vi "File Page - Set Stop Trigger.vi"(7 "File Ctl Refs":T3, 8 "error in (no error)":errorcluster, 10 "Stop Trigger":T1 caption="Trigger condition", 11 "Item Ref in":T2 format="%.0x") -> (0 "error out":errorcluster)   [LabVIEW 2015, in "Waveform Data Logger System Explorer.lvlib"]
uses:
  Waveform Data Logger System Explorer.lvlib
  Types/File Ctl Refs.ctl
  Types/File - Spec Ctl Refs.ctl
  Types/File - Wfm Ctl Refs.ctl
  Types/File - Settings Ctl Refs.ctl
  Classes/Log File Specifications/Log File Specification/File Conflict Operation.ctl
  Types/File - Start Trig Ctl Refs.ctl
  Shared/Types/Start Trigger.ctl
  Shared/Types/Default Trigger.ctl
  Shared/Types/Digital Trigger.ctl
  Shared/Types/Analog Trigger.ctl
  Shared/Types/In Range Trigger.ctl
  Shared/Types/Value Change Trigger.ctl
  Shared/Types/Boolean Trigger.ctl
  Types/Single Node Browser Data.ctl
  <vilib>/NI Veristand/UI Controls/Single Node Browser/Single Node Browser Ref.ctl
  NationalInstruments.VeriStand.SystemStorageUI
  <vilib>/NI Veristand/UI Controls/Single Node Browser/Callback Type.ctl
  <vilib>/NI Veristand/UI Controls/Single Node Browser/Net Event Data.ctl
  <vilib>/NI Veristand/UI Controls/Single Node Browser/Net Event.ctl
  Types/File - Stop Trig Ctl Refs.ctl
  Shared/Types/Stop Trigger.ctl
  Types/File - Advanced Ctl Refs.ctl
  Types/Log Timestamps.ctl
  <vilib>/NI Veristand/Custom Device API/Custom Device Item Ref.ctl
  NationalInstruments.VeriStand.SystemStorage
  Shared/Globals/Property Strings.vi
  <vilib>/NI Veristand/Custom Device API/Set Item Property (U16).vi
  <vilib>/NI Veristand/Custom Device API/Get Item Property (Dependent Node Pointer).vi
  <vilib>/NI Veristand/Custom Device API/Set Item Property (Dependent Node Pointer).vi
  <vilib>/NI Veristand/Custom Device API/Custom Device API.lvlib
  Shared/Waveform Data Logger Shared.lvlib
  Classes/Log File Specifications/Log File Specification/Log File Specification.lvclass
  <vilib>/NI Veristand/UI Controls/Single Node Browser/NI_VS UI Single Node Browser.lvlib
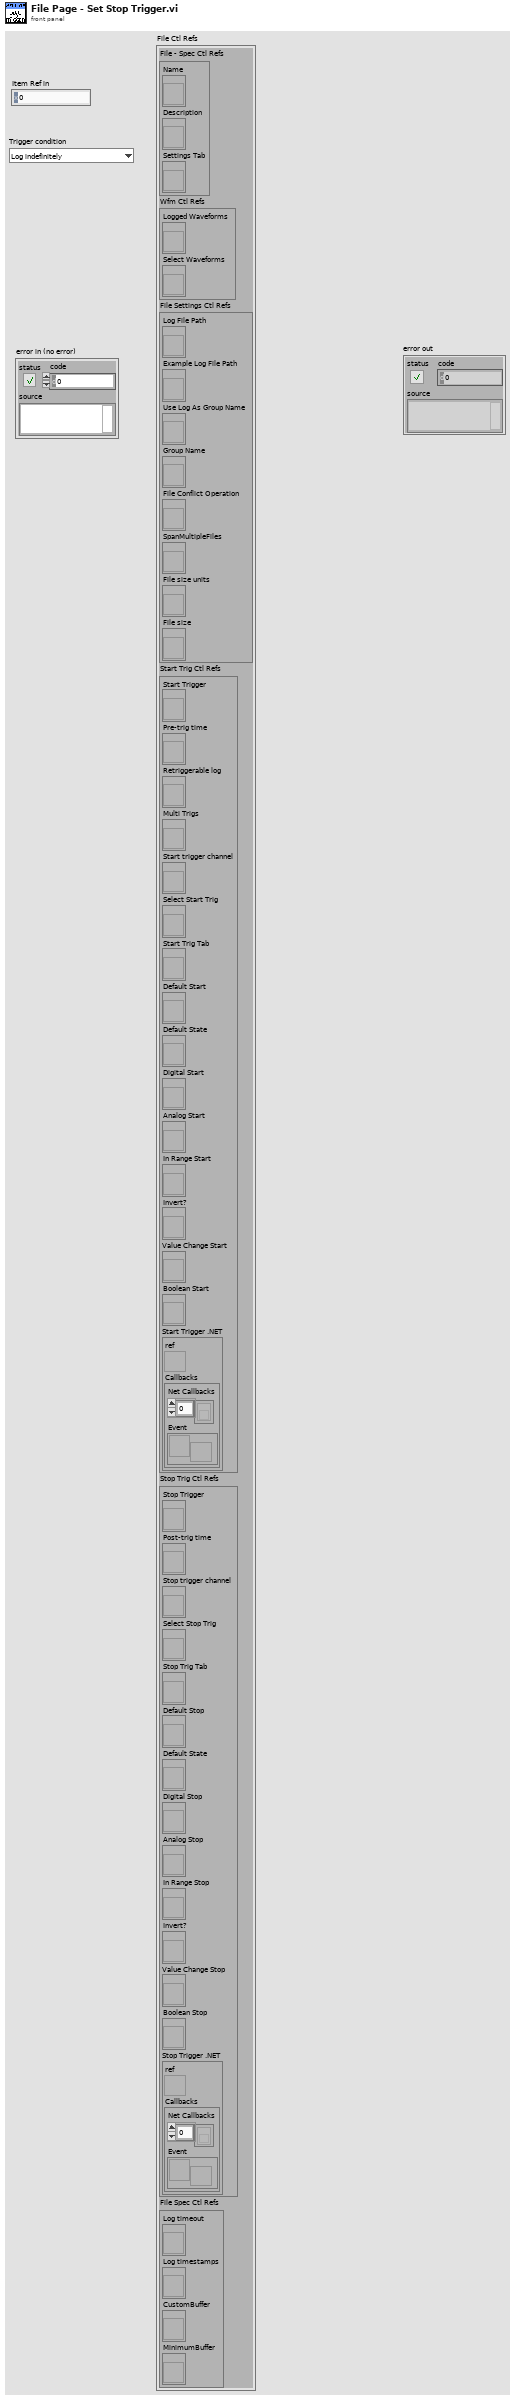
[diagram p1: front panel]
types:
  T1 = typedef "Waveform Data Logger Shared.lvlib/Stop Trigger.ctl" = enum16{"Log indefinitely", "Stop after duration", "Stop on digital edge", "Stop on analog edge", "Stop when in range", "Stop when out of range", "Stop on value change", "Stop when Boolean condition is true"}
  T2 = typedef "Custom Device API.lvlib/Custom Device Item Ref.ctl" = u64
  T3 = typedef "Waveform Data Logger System Explorer.lvlib/File Ctl Refs.ctl" = cluster{"File Spec Ctl Refs":T4, "Wfm Ctl Refs":T5, "File Settings Ctl Refs":T6, "Start Trig Ctl Refs":T7, "Stop Trig Ctl Refs":T11, "File Spec Ctl Refs":T12}
  T4 = typedef "Waveform Data Logger System Explorer.lvlib/File - Spec Ctl Refs.ctl" = cluster{"Name":refnum<vi>, "Description":refnum<vi>, "Settings Tab":refnum<vi>}
  T5 = typedef "Waveform Data Logger System Explorer.lvlib/File - Wfm Ctl Refs.ctl" = cluster{"Logged Waveforms":refnum<vi>, "Select Waveforms":refnum<vi>}
  T6 = typedef "Waveform Data Logger System Explorer.lvlib/File - Settings Ctl Refs.ctl" = cluster{"Log File Path":refnum<vi>, "Example Log File Path":refnum<vi>, "Use Log As Group Name":refnum<vi>, "Group Name":refnum<vi>, "File Conflict Operation":refnum<vi>, "SpanMultipleFiles":refnum<vi>, "File size units":refnum<vi>, "File size":refnum<vi>}
  T7 = typedef "Waveform Data Logger System Explorer.lvlib/File - Start Trig Ctl Refs.ctl" = cluster{"Start Trigger":refnum<vi>, "Pre-trig time":refnum<vi>, "Retriggerable log":refnum<vi>, "Multi Trigs":refnum<vi>, "Start trigger channel":refnum<vi>, "Select Start Trig":refnum<vi>, "Start Trig Tab":refnum<vi>, "Default Start":refnum<vi>, "Default State":refnum<vi>, "Digital Start":refnum<vi>, "Analog Start":refnum<vi>, "In Range Start":refnum<vi>, "Invert?":refnum<vi>, "Value Change Start":refnum<vi>, "Boolean Start":refnum<vi>, "Start Trigger .NET":T8}
  T8 = typedef "Waveform Data Logger System Explorer.lvlib/Single Node Browser Data.ctl" = cluster{"ref":T9, "Callbacks":T10}
  T9 = typedef "NI_VS UI Single Node Browser.lvlib/Single Node Browser Ref.ctl" = refnum<k24>
  T10 = typedef "NI_VS UI Single Node Browser.lvlib/Callback Type.ctl" = cluster{"Net Callbacks":refnum<k27>[], "Event":refnum<user-event>}
  T11 = typedef "Waveform Data Logger System Explorer.lvlib/File - Stop Trig Ctl Refs.ctl" = cluster{"Stop Trigger":refnum<vi>, "Post-trig time":refnum<vi>, "Stop trigger channel":refnum<vi>, "Select Stop Trig":refnum<vi>, "Stop Trig Tab":refnum<vi>, "Default Stop":refnum<vi>, "Default State":refnum<vi>, "Digital Stop":refnum<vi>, "Analog Stop":refnum<vi>, "In Range Stop":refnum<vi>, "Invert?":refnum<vi>, "Value Change Stop":refnum<vi>, "Boolean Stop":refnum<vi>, "Stop Trigger .NET":T8}
  T12 = typedef "Waveform Data Logger System Explorer.lvlib/File - Advanced Ctl Refs.ctl" = cluster{"Log timeout":refnum<vi>, "Log timestamps":refnum<vi>, "CustomBuffer":refnum<vi>, "MinimumBuffer":refnum<vi>}
  T13 = enum32{"Default", "Digital", "Analog", "In Range", "Value Change", "Boolean"}
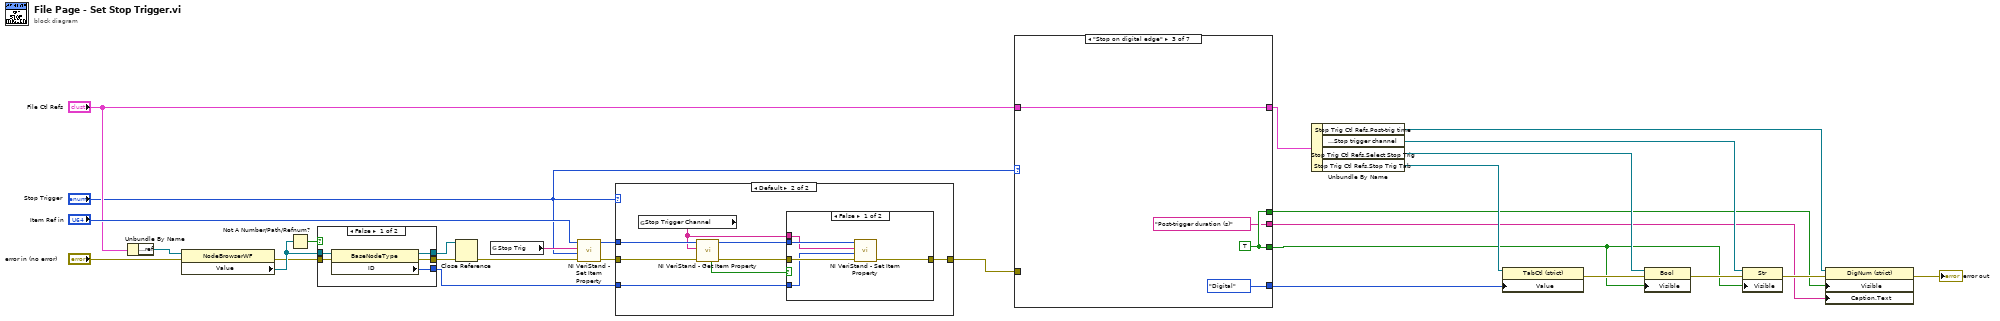
[diagram p0: block diagram]
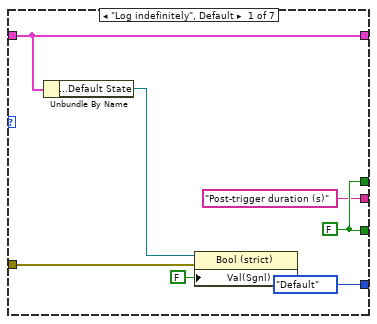
[diagram p2: hidden frame]
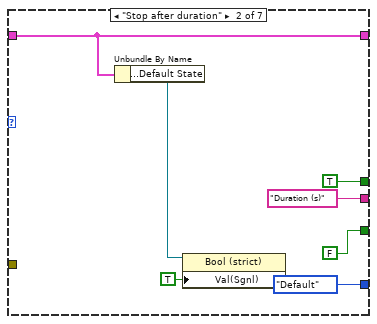
[diagram p3: hidden frame]
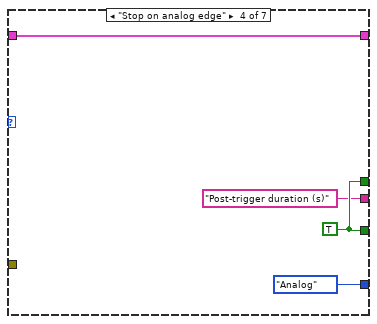
[diagram p4: hidden frame]
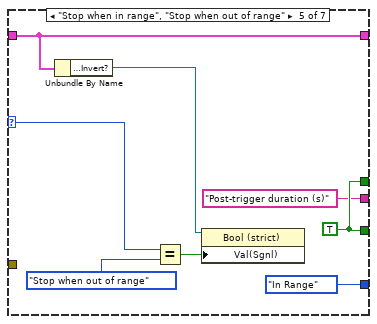
[diagram p5: hidden frame]
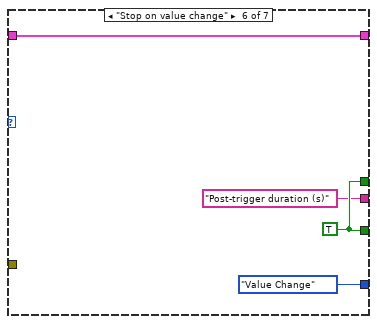
[diagram p6: hidden frame]
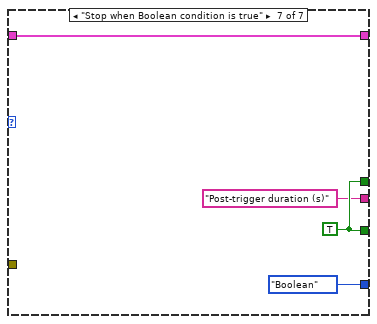
[diagram p7: hidden frame]
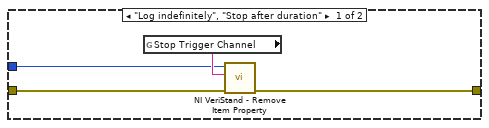
[diagram p8: hidden frame]
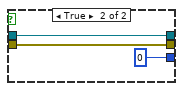
[diagram p10: hidden frame]
diagram:
  n1 = Unbundle By Name("File Ctl Refs") -> ("Stop Trig Ctl Refs.Stop Trigger .NET.ref"=w28:T9)
  n2 = property class="NodeBrowserWF"(reference=w28, error in="error in (no error)") -> (error out=w25:errorcluster, "Value"=w26:refnum<k24>)  [unwired: 1 out]
  n3 = Not A Number/Path/Refnum?(number/path/refnum=w26) -> (NaN/Path/Refnum?=w27:bool)
  n4 = case shown="False" w27 {
    tunnel: [w34 u64 0 ("ID")] -> w17
    tunnel: w25 -> [w33 w37]
    tunnel: [w30 w37] -> w24
    tunnel: w26 -> [w32 w35]
    tunnel: [w31 w35] -> w23
    frame False {
      n5 = property class="BaseNodeType"(reference=w32, error in=w33) -> (reference out=w31:refnum<k24>, error out=w30:errorcluster, "ID"=w34:u64)
    }
    frame True {
    }
  }
  n6 = Close Reference(reference=w23, error in (no error)=w24) -> (error out=w21:errorcluster)
  n7 = global read "Property Strings.vi" "Stop Trig"() -> (w22:string)
  n8 = call-poly <vilib>:"NI VeriStand - Set Item Property.vi"("error in (no error)"=w21, "Value"="Stop Trigger", "Property Name"=w22, "Item Ref in"="Item Ref in") -> ("error out"=w18:errorcluster, "Item Ref out"=w19:T2)  [unwired: 5 in, 1 out]
  n9 = case shown="Default" "Stop Trigger" {
    tunnel: w18 -> [w40 w47]
    tunnel: w19 -> [w39 w48]
    tunnel: [w38 w49] -> w15
    tunnel: w17 -> [_ w42]
    frame "Log indefinitely", "Stop after duration" {
      n10 = global read "Property Strings.vi" "Stop Trigger Channel"() -> (w41:string)
      n11 = call <vilib>:"NI VeriStand - Remove Item Property.vi"("error in (no error)"=w40, "Property Name"=w41, "Item Ref in"=w39) -> ("error out"=w38:errorcluster)  [unwired: 6 in, 2 out]
    }
    frame Default {
      n12 = global read "Property Strings.vi" "Stop Trigger Channel"() -> (w43:string)
      n13 = call-poly <vilib>:"NI VeriStand - Get Item Property.vi"("error in (no error)"=w47, "Property Name"=w43, "Item Ref in"=w48) -> ("error out"=w45:errorcluster, "Item Ref out"=w44:T2, "Found"=w46:bool)  [unwired: 6 out]
      n14 = case shown="False" w46 {
        tunnel: [w54 w55] -> w49
        tunnel: w45 -> [w53 w55]
        tunnel: w44 -> [w52 _]
        tunnel: w43 -> [w51 _]
        tunnel: w42 -> [w50 _]
        frame False {
          n15 = call-poly <vilib>:"NI VeriStand - Set Item Property.vi"("error in (no error)"=w53, "Dependent Node Ref"=w50, "Property Name"=w51, "Item Ref in"=w52) -> ("error out"=w54:errorcluster)  [unwired: 7 out]
        }
        frame True {
        }
      }
    }
  }
  n16 = case shown="\"Stop on digital edge\"" "Stop Trigger" {
    selector: "Stop Trigger" -> [_ _ _ _ w81 _ _]
    tunnel: [w61 FALSE w72 w76 w84 w88 w92] -> w6
    tunnel: [T13."Default" ("Start Trig Tab") T13."Default" ("Start Trig Tab") T13."Digital" ("Start Trig Tab") T13."Analog" ("Start Trig Tab") T13."In Range" ("Start Trig Tab") T13."Value Change" ("Start Trig Tab") T13."Boolean" ("Start Trig Tab")] -> w11
    tunnel: [w61 TRUE w72 w76 w84 w88 w92] -> w3
    tunnel: ["Post-trigger duration (s)" "Duration (s)" "Post-trigger duration (s)" "Post-trigger duration (s)" "Post-trigger duration (s)" "Post-trigger duration (s)" "Post-trigger duration (s)"] -> w2
    tunnel: "File Ctl Refs" -> [w58 w64 w70 w74 w79 w86 w90]
    tunnel: [w58 w64 w70 w74 w79 w86 w90] -> w13
    tunnel: w15 -> [w56 _ _ _ _ _ _]
    frame "Log indefinitely", Default {
      w61 = FALSE
      n17 = Unbundle By Name(w58) -> ("Stop Trig Ctl Refs.Default State"=w57:refnum<vi>)
      n18 = property on="Property Node" class="Bool (strict)"(reference=w57, error in=w56, "Val(Sgnl)"=FALSE ("Visible")) -> ()  [unwired: 2 out]
    }
    frame "Stop after duration" {
      n19 = Unbundle By Name(w64) -> ("Stop Trig Ctl Refs.Default State"=w63:refnum<vi>)
      n20 = property on="Property Node" class="Bool (strict)"(reference=w63, "Val(Sgnl)"=TRUE ("Visible")) -> ()  [unwired: 1 in, 2 out]
    }
    frame "Stop on digital edge" {
      w72 = TRUE
    }
    frame "Stop on analog edge" {
      w76 = TRUE
    }
    frame "Stop when in range", "Stop when out of range" {
      w84 = TRUE
      n21 = Unbundle By Name(w79) -> ("Stop Trig Ctl Refs.Invert?"=w78:refnum<vi>)
      n22 = Equal?(x=w81, y=Stop_Trigger."Stop when out of range" ("Stop Trigger")) -> (x = y?=w82:bool)
      n23 = property on="Property Node" class="Bool (strict)"(reference=w78, "Val(Sgnl)"=w82) -> ()  [unwired: 1 in, 2 out]
    }
    frame "Stop on value change" {
      w88 = TRUE
    }
    frame "Stop when Boolean condition is true" {
      w92 = TRUE
    }
  }
  n24 = Unbundle By Name(w13) -> ("Stop Trig Ctl Refs.Post-trig time"=w4:refnum<vi>, "Stop Trig Ctl Refs.Stop trigger channel"=w7:refnum<vi>, "Stop Trig Ctl Refs.Select Stop Trig"=w9:refnum<vi>, "Stop Trig Ctl Refs.Stop Trig Tab"=w12:refnum<vi>)
  n25 = property class="TabCtl (strict)"(reference=w12, "Value"=w11) -> (error out=w10:errorcluster)  [unwired: 1 in, 1 out]
  n26 = property class="Bool"(reference=w9, error in=w10, "Visible"=w6) -> (error out=w8:errorcluster)  [unwired: 1 out]
  n27 = property class="Str"(reference=w7, error in=w8, "Visible"=w6) -> (error out=w5:errorcluster)  [unwired: 1 out]
  n28 = property on="Property Node" class="DigNum (strict)"(reference=w4, error in=w5, "Visible"=w3, "Caption.Text"=w2) -> (error out=→"error out":errorcluster)  [unwired: 1 out]
